vi "Run Script.vi"(8 "error in (no error)":errorcluster, 10 "Script Path":path, 11 "BFECC in":refnum<class "BFECC.lvclass">) -> (0 "error out":errorcluster, 3 "BFECC out":refnum<class "BFECC.lvclass">)   [LabVIEW 2018, in "BFECC.lvlib" / "BFECC.lvclass"]
uses:
  BFECC.lvclass
  BFECC.lvclass/BFECC.ctl
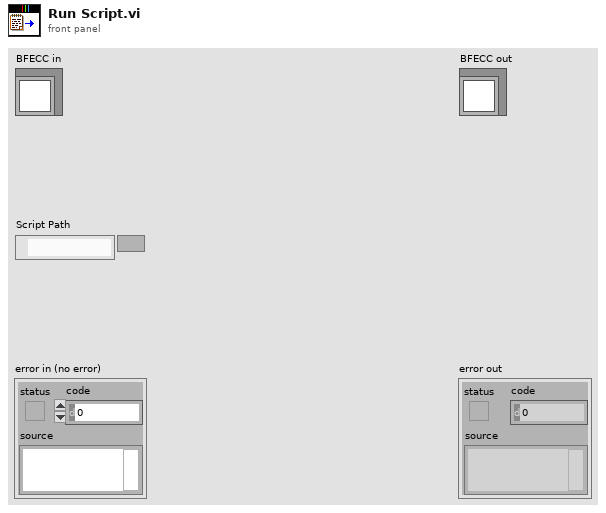
[diagram p1: front panel]
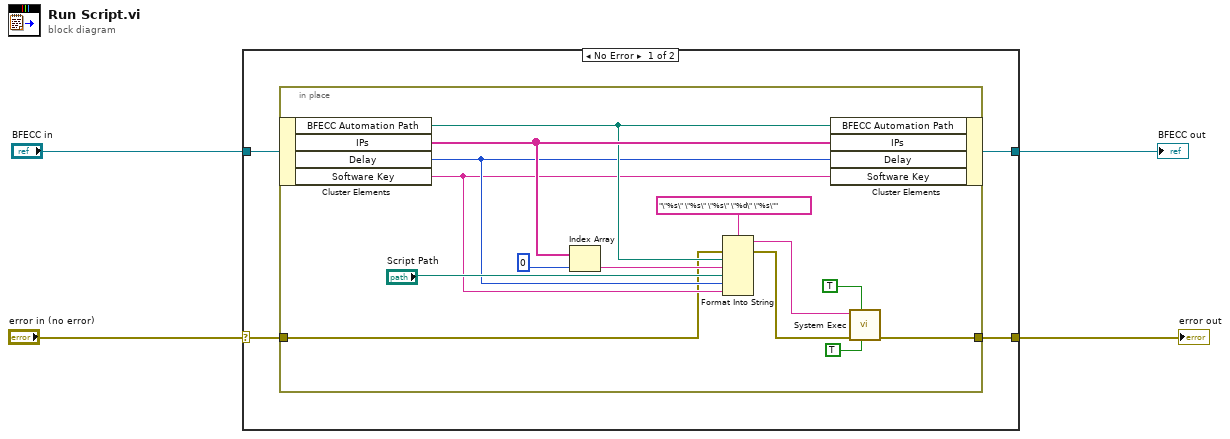
[diagram p0: block diagram]
diagram:
  n1 = case shown="No Error" "error in (no error)" {
    selector: "error in (no error)" -> [w7 w24]
    tunnel: [w5 w24] -> w3
    tunnel: [w6 w23] -> w1
    tunnel: "BFECC in" -> [w8 w23]
    frame No Error {
      n2 = in-place {
        in-place-border: w7 -> [w14]
        in-place-border: [w12] -> w5
        n3 = in-place-cluster #1(w8) -> ("BFECC Automation Path"=w19:path, "IPs"=w21:string[], "Delay"=w16:u32, "Software Key"=w15:string)
        n4 = Index Array(array=w21, index=0) -> (element=w18:string)
        n5 = Format Into String(format string="\"%s\" \"%s\" \"%s\" \"%d\" \"%s\"", error in=w14, w19, w18, "Script Path", w16, w15) -> (resulting string=w11:string, error out=w13:errorcluster)  [unwired: 1 in]
        n6 = in-place-cluster #1("BFECC Automation Path"=w19, "IPs"=w21, "Delay"=w16, "Software Key"=w15) -> (w6:refnum<class "BFECC.lvclass">)
        n7 = call <vilib>:"System Exec.vi"("run minimized? (F)"=TRUE, "wait until completion? (T)"=TRUE, "error in (no error)"=w13, "command line"=w11) -> ("error out"=w12:errorcluster)  [unwired: 4 in, 3 out]
      }
    }
    frame Error {
    }
  }
  "error out" <- w3
  "BFECC out" <- w1
